vi "Read Config File.vi"(8 "error in (no error)":errorcluster, 11 "Trace Grabber Application in":refnum<class "User Interface.lvclass">) -> (0 "error out":errorcluster, 3 "Trace Grabber Application out":refnum<class "User Interface.lvclass">)   [LabVIEW 2016, in "User Interface.lvlib" / "User Interface.lvclass"]
uses:
  User Interface.lvclass
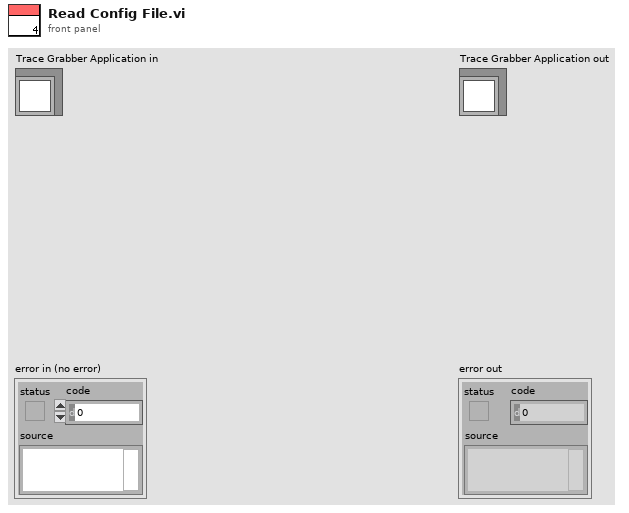
[diagram p1: front panel]
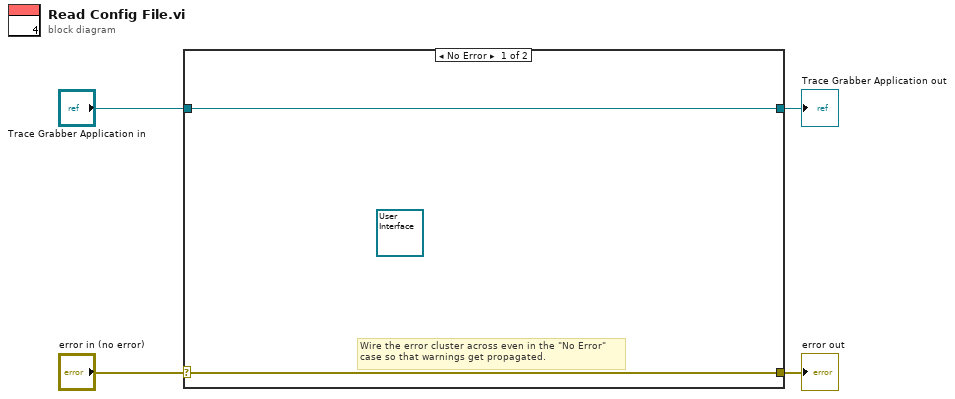
[diagram p0: block diagram]
diagram:
  n1 = case shown="No Error" "error in (no error)" {
    selector: "error in (no error)" -> [w5 w8]
    tunnel: [w5 w8] -> w3
    tunnel: [w6 w7] -> w1
    tunnel: "Trace Grabber Application in" -> [w6 w7]
    frame No Error {
      (unwired) refnum<class "User Interface.lvclass"> refnum ("Trace Grabber Application.lvlib:Trace Grabber Application.lvclass")
      # "Wire the error cluster across even in the \"No Error\"\ncase so that warnings get propagated."
    }
    frame Error {
    }
  }
  "error out" <- w3
  "Trace Grabber Application out" <- w1
